vi "Wait-Stop-Buttton.vi"(8 "Error In":errorcluster) -> (0 "Error Out":errorcluster)   [LabVIEW 2019]
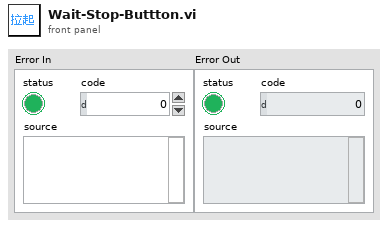
[diagram p1: front panel]
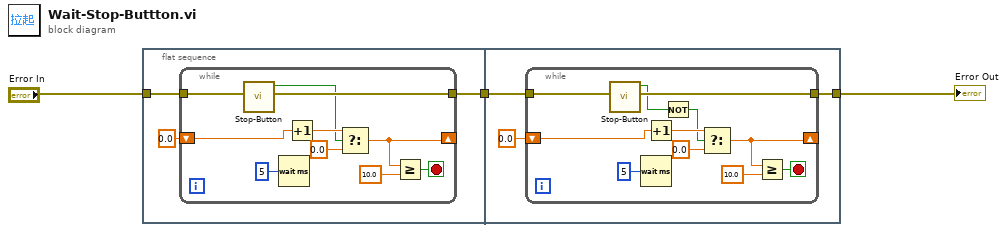
[diagram p0: block diagram]
diagram:
  n1 = flat-sequence {
    tunnel: "Error In" -> [w6]
    tunnel: [w5] -> w3
    tunnel: w3 -> [w17]
    tunnel: [w18] -> w1
    frame #0 {
      n2 = while {
        tunnel: w6 -> [w7]
        tunnel: [w9] -> w5
        shift-right: [w11] -> _
        shift-left: 0.0 -> [w14]
        stop <- w12 stop-if-true
        n3 = call "Stop-Button.vi"("Error In"=w7) -> ("Error Out"=w9:errorcluster, "顯示按下?"=w8:bool)  [unwired: 9 in]
        n4 = Wait (ms)(milliseconds to wait=u32 5) -> ()  [unwired: 1 out]
        n5 = Increment(x=w14) -> (x+1=w15:dbl)
        n6 = Select(t=w15, s=w8, f=0.0) -> (s? t:f=w11:dbl)
        n7 = Greater Or Equal?(x=w11, y=10.0) -> (x >= y?=w12:bool)
      }
    }
    frame #1 {
      n8 = while {
        tunnel: w17 -> [w21]
        tunnel: [w22] -> w18
        shift-right: [w25] -> _
        shift-left: 0.0 -> [w28]
        stop <- w26 stop-if-true
        n9 = call "Stop-Button.vi"("Error In"=w21) -> ("Error Out"=w22:errorcluster, "顯示按下?"=w20:bool)  [unwired: 9 in]
        n10 = Wait (ms)(milliseconds to wait=u32 5) -> ()  [unwired: 1 out]
        n11 = Increment(x=w28) -> (x+1=w29:dbl)
        n12 = Not(x=w20) -> (.not. x?=w23:bool)
        n13 = Select(t=w29, s=w23, f=0.0) -> (s? t:f=w25:dbl)
        n14 = Greater Or Equal?(x=w25, y=10.0) -> (x >= y?=w26:bool)
      }
    }
  }
  "Error Out" <- w1
